vi "ProcessCoin.vi"(8 "error in (no error)":errorcluster, 10 "USD Coin":cluster{"1":bool, "2":bool, "3":bool}, 11 "USD Actor in":refnum<class "USD Actor.lvclass">) -> (0 "error out":errorcluster, 3 "USD Actor out":refnum<class "USD Actor.lvclass">)   [LabVIEW 2020, in "USD Actor.lvlib" / "USD Actor.lvclass"]
uses:
  USD Actor.lvclass
  C:/Program Files (x86)/National Instruments/LabVIEW 2020/vi.lib/ActorFramework/Actor/Actor.lvclass
  <vilib>/ActorFramework/Actor/Actor.lvclass/Actor.ctl
  USD Actor.lvclass/USD Actor.ctl
  UI Actor Messages/creditUpdate Msg/creditUpdate Msg.lvclass/creditUpdate Msg.ctl
  <vilib>/ActorFramework/Message Enqueuer/Message Enqueuer.lvclass/Message Enqueuer.ctl
  <vilib>/ActorFramework/Message Enqueuer/Enqueue.vi
  UI Actor Messages/creditUpdate Msg/creditUpdate Msg.lvclass
  C:/Program Files (x86)/National Instruments/LabVIEW 2020/vi.lib/ActorFramework/Message/Message.lvclass
  <vilib>/ActorFramework/Message Priority Queue/Priority Enqueue.vi
  <vilib>/ActorFramework/Actor/Actor.lvclass
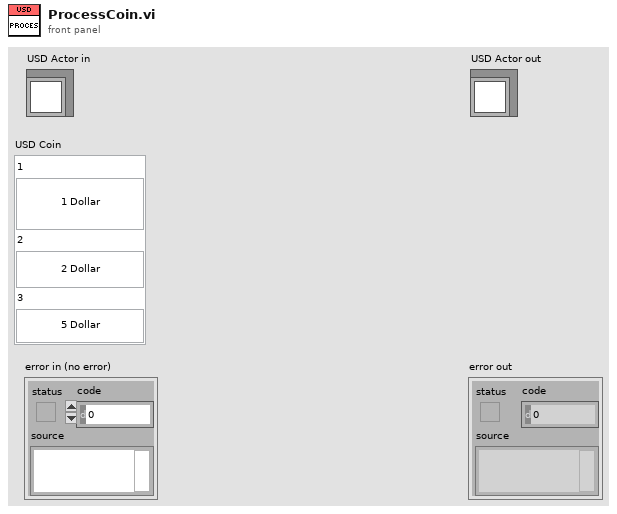
[diagram p1: front panel]
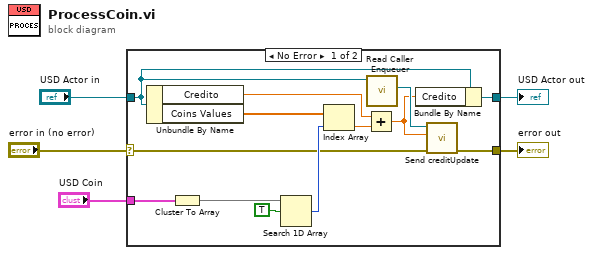
[diagram p0: block diagram]
diagram:
  n1 = case shown="No Error" "error in (no error)" {
    selector: "error in (no error)" -> [w7 w20]
    tunnel: [w6 w20] -> w4
    tunnel: [w12 w19] -> w2
    tunnel: "USD Actor in" -> [w10 w19]
    tunnel: "USD Coin" -> [w11 _]
    frame No Error {
      n2 = Unbundle By Name(w10) -> ("Credito"=w13:dbl, "Coins Values"=w16:dbl[])
      n3 = Cluster To Array(cluster=w11) -> (array=w18:bool[])
      n4 = Search 1D Array(1D array=w18, element=TRUE) -> (index of element=w15:i32)  [unwired: 1 in]
      n5 = Index Array(array=w16, index=w15) -> (element=w14:dbl)
      n6 = Add(x=w13, y=w14) -> (x+y=w8:dbl)
      n7 = call <vilib>:"Read Caller Enqueuer.vi"("Actor"=w10) -> ("Caller Enqueuer"=w9:refnum<class "Message Enqueuer.lvclass">)  [unwired: 10 in]
      n8 = Bundle By Name(cluster=w10, "Credito"=w8) -> (w12:refnum<class "USD Actor.lvclass">)
      n9 = call "Send creditUpdate.vi"("error in (no error)"=w7, "Credit"=w8, "Message Enqueuer"=w9) -> ("error out"=w6:errorcluster)  [unwired: 7 in, 1 out]
    }
    frame Error {
    }
  }
  "error out" <- w4
  "USD Actor out" <- w2
